vi "startcase2.vi"() -> ()   [LabVIEW 2015]
panel:
  out "String 2":string
  in  "String":string
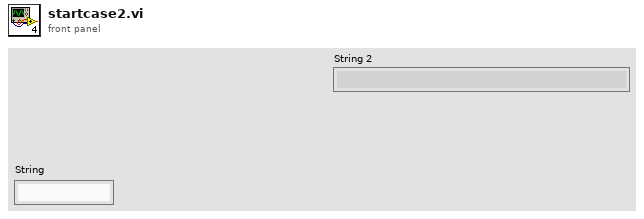
[diagram p1: front panel]
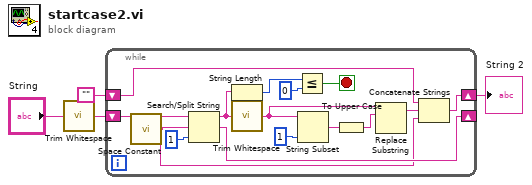
[diagram p0: block diagram]
diagram:
  n1 = call <vilib>:"Trim Whitespace.vi"("string"="String") -> ("trimmed string"=w3:string)  [unwired: 1 in]
  n2 = while {
    shift-right: [w7] -> w1
    shift-left: "" -> [w8]
    shift-right: [w16] -> _
    shift-left: w3 -> [w17]
    stop <- w18 stop-if-true
    n3 = call <vilib>:"Space Constant.vi"() -> ("String"=w5:string)
    n4 = Search/Split String(string=w17, search string/char (-)=w5, offset (0)=1) -> (substring before match=w14:string, match + rest of string=w16:string)  [unwired: 1 out]
    n5 = String Length(string=w14) -> (length=w10:i32)
    n6 = call <vilib>:"Trim Whitespace.vi"("string"=w14) -> ("trimmed string"=w12:string)  [unwired: 1 in]
    n7 = Less Or Equal?(x=w10, y=0) -> (x <= y?=w18:bool)
    n8 = String Subset(string=w12, length (rest)=1 ("y")) -> (substring=w13:string)  [unwired: 1 in]
    n9 = To Upper Case(1:w13) -> (0:w11:string)
    n10 = Replace Substring(4:w11, 5:w12) -> (1:w6:string)  [unwired: 2 in, 1 out]
    n11 = Concatenate Strings(w8, w6, w5) -> (w7:string)
  }
  "String 2" <- w1
